vi "About Dialog.vi"(8 "error in (no error)":errorcluster, 11 "SW Version":string) -> (0 "error out":errorcluster)   [LabVIEW 2014, in "Raspberry Pi Compatible Compiler for LabVIEW.lvlib"]
doc: "About Dialog Box."
uses:
  Raspberry Pi Compatible Compiler for LabVIEW.lvlib
panel:
  in  "OK":bool
  out "Version":string
  # "© 2016 TSXperts LLC\n© 2016 SpoolWerks.\nAll Rights Reserved."
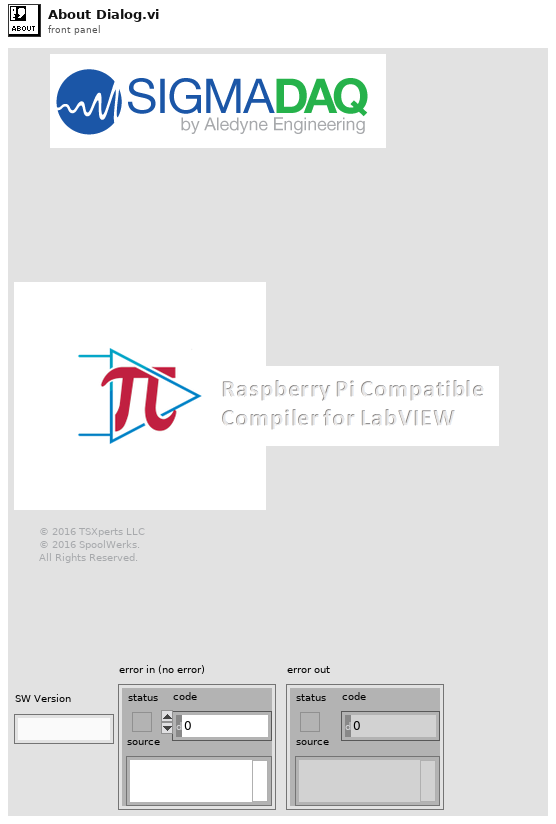
[diagram p1: front panel]
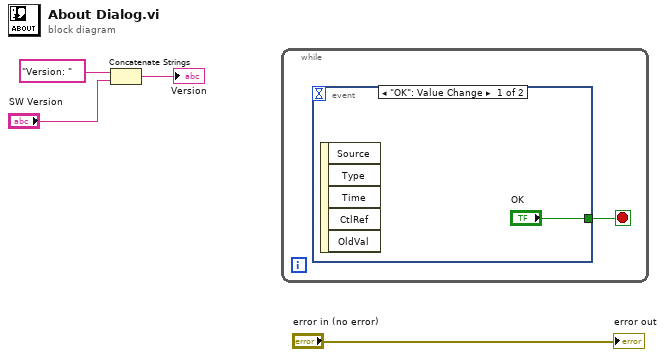
[diagram p0: block diagram]
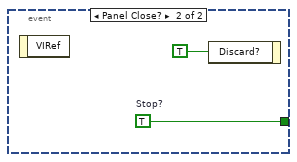
[diagram p2: hidden frame]
diagram:
  n1 = Concatenate Strings("Version: " ("string"), "SW Version") -> (→"Version":string)
  n2 = while {
    stop <- w5 stop-if-true
    n3 = event shown="[0] \"OK\": Value Change" {
      selector: _ -> [_ _]
      dyn-events: _ -> [_ _]
      timeout: _ -> [_ _]
      tunnel: ["OK" w7] -> w5
      event "OK": Value Change {
        n4 = event-data() -> ()  [unwired: 6 out]
      }
      event Panel Close? {
        w7 = TRUE  # Stop?
        n5 = event-data() -> ()  [unwired: 2 out]
        n6 = event-data("Discard?"=TRUE) -> ()  [unwired: 1 in, 1 out]
      }
    }
  }
  "error out" <- "error in (no error)"
